vi "Teleop.vi"(10 "Match Info":T1={"Autonomous Elapsed Seconds"=0.0, "TeleOp Elapsed Seconds"=0.0, "Disabled Elapsed Seconds"=0.0, "Visited Autonomous"=FALSE, "Visited TeleOp"=FALSE, "Visited Disabled"=FALSE, "Autonomous Settings"={"Autonomous Style"=enum."Independent", "VI Refnum"=refnum}}, 11 "Call Context":T2) -> ()   [LabVIEW 2012]
doc: "This VI is called for each TeleOp packet received from the DS where the robot is not disabled. It is often used to read from the joysticks and update I/O or to update setpoints for timed control loops. It should complete and return within 20 milliseconds or it may miss DS packets."
uses:
  <vilib>/Rock Robotics/WPI/DriverStation/WPI_DriverStationDerivedRobotMode.ctl
  <vilib>/Rock Robotics/WPI/DriverStation/WPI_DriverStationMatch Info.ctl
  <vilib>/Rock Robotics/WPI/Relay/WPI_RelayValue.ctl
  Robot Global Data.vi
  <vilib>/Rock Robotics/WPI/Joystick/WPI_JoystickGetSetRefNum.vi
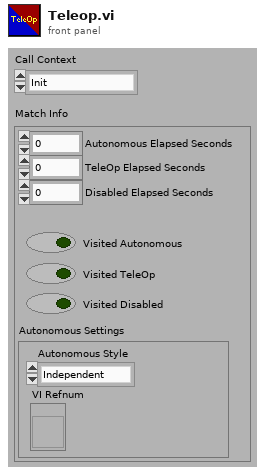
[diagram p1: front panel]
types:
  T1 = typedef "WPI_DriverStationMatch Info.ctl" = cluster{"Autonomous Elapsed Seconds":dbl, "TeleOp Elapsed Seconds":dbl, "Disabled Elapsed Seconds":dbl, "Visited Autonomous":bool, "Visited TeleOp":bool, "Visited Disabled":bool, "Autonomous Settings":cluster{"Autonomous Style":enum16{"Iterative", "Independent"}, "VI Refnum":refnum<vi>}}
  T2 = typedef "WPI_DriverStationDerivedRobotMode.ctl" = enum16{"Init", "Execute", "Stop"}
  T3 = typedef "WPI_JoystickDevRef.ctl" = cluster{"Device":T4}
  T4 = typedef "WPI_JoystickDeviceEnum.ctl" = enum16{"USB 1", "USB 2", "USB 3", "USB 4", "Kinect 1", "Kinect 2"}
  T5 = typedef "WPI_JoystickButtonState.ctl" = cluster{"Button 1":bool, "Button 2":bool, "Button 3":bool, "Button 4":bool, "Button 5":bool, "Button 6":bool, "Button 7":bool, "Button 8":bool, "Button 9":bool, "Button 10":bool, "Button 11":bool, "Button 12":bool}
  T6 = cluster{"axis 1 (x)":dbl, "axis 2 (y)":dbl, "axis 3 (throttle)":dbl, "axis 4":dbl, "axis 5":dbl, "axis 6":dbl}
  T7 = typedef "WPI_RelayValue.ctl" = enum16{"Off", "On", "Forward", "Reverse"}
  T8 = typedef "WPI_MotorControlDeviceRef.ctl" = cluster{"DeviceStatus":errorcluster, "Type":enum16{"PWM", "CAN"}, "PWM":cluster{"Digital Module":T9, "PWM Channel":T10, "DeadBand":T11}, "CAN":cluster{"Device Number":u8, "Control Mode":T12, "Semaphore":T13, "Max Vout":dbl}, "Invert":bool, "TransformRef":T14, "InvTransformRef":T14}
  T9 = typedef "FPGA_TypedefDigitalModule.ctl" = enum16{"Digital Module 1", "Digital Module 2"}
  T10 = typedef "FPGA_DIOPWMChannel.ctl" = enum8{"PWM 1", "PWM 2", "PWM 3", "PWM 4", "PWM 5", "PWM 6", "PWM 7", "PWM 8", "PWM 9", "PWM 10", "Invalid"}
  T11 = typedef "WPI_PWMDeadband.ctl" = cluster{"Name":string, "maxPositivePwm":i32, "minPositivePwm":i32, "centerPwm":i32, "maxNegativePwm":i32, "minNegativePwm":i32, "angularRange":u16}
  T12 = typedef "WPI_CANJaguar_ControlMode.ctl" = enum8{"Percent VBus", "Current", "Speed", "Position", "Voltage"}
  T13 = typedef "Semaphore RefNum" = refnum<k1>
  T14 = typedef "WPI_PWMTransform_ConPane.ctl" = refnum<vi>
  T15 = typedef "WPI_RelayDevRef.ctl" = cluster{"DevStatus":errorcluster, "Relay Channel":T16, "Digital Module":T9, "Relay Direction":T17}
  T16 = typedef "FPGA_DIORelayChannel.ctl" = enum8{"Relay 1", "Relay 2", "Relay 3", "Relay 4", "Relay 5", "Relay 6", "Relay 7", "Relay 8", "Invalid"}
  T17 = typedef "WPI_RelayDirection.ctl" = enum16{"Both directions", "Forward only", "Reverse only"}
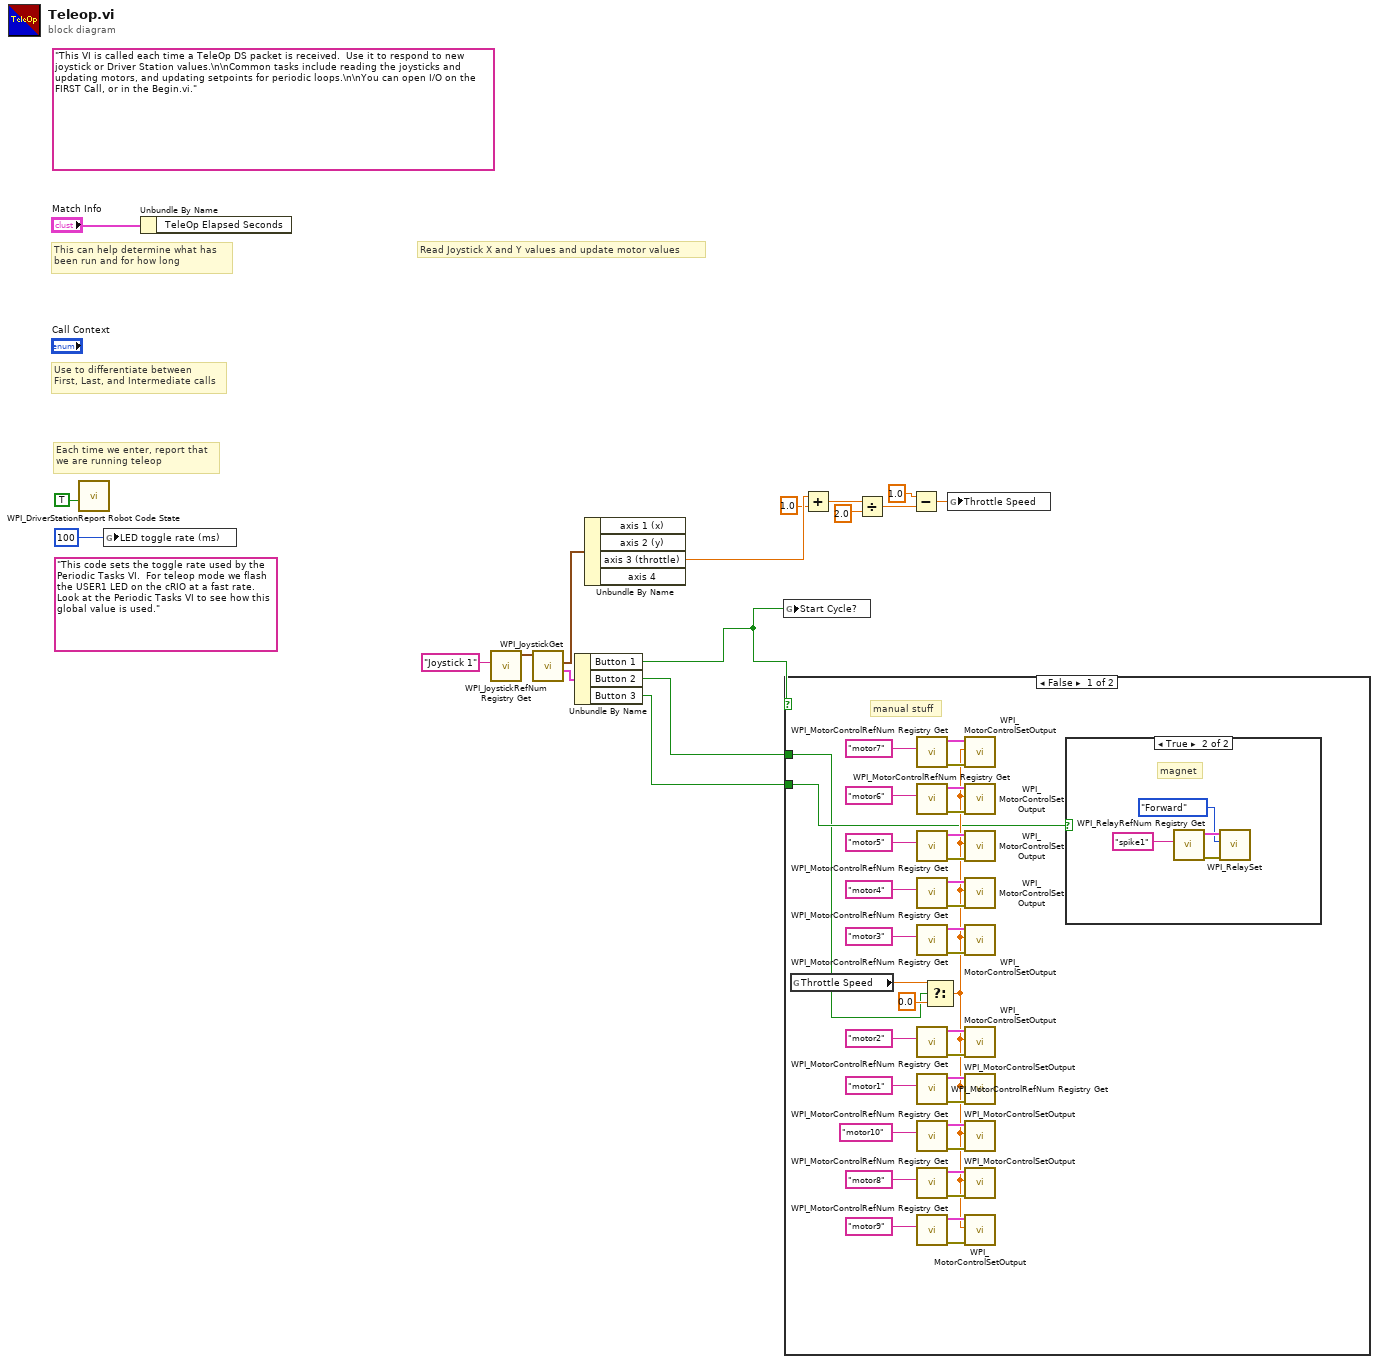
[diagram p0: block diagram]
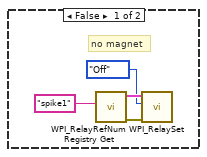
[diagram p2: hidden frame]
diagram:
  (unwired) "This code sets the toggle rate used by the Periodic Tasks VI.  For teleop mode we flash the USER1 LED on the cRIO at a fast rate.  Look at the Periodic Tasks VI to see how this global value is used."
  (unwired) "This VI is called each time a TeleOp DS packet is received.  Use it to respond to new joystick or Driver Station values.\n\nCommon tasks include reading the joysticks and updating motors, and updating setpoints for periodic loops.\n\nYou can open I/O on the FIRST Call, or in the Begin.vi."
  # "Each time we enter, report that\nwe are running teleop"
  # "Use to differentiate between\nFirst, Last, and Intermediate calls"
  # "This can help determine what has\nbeen run and for how long"
  # "Read Joystick X and Y values and update motor values"
  n1 = call <vilib>:"WPI_DriverStationReport Robot Code State.vi"("TeleOp"=TRUE ("Autonomous")) -> ()  [unwired: 10 in, 1 out]
  n2 = global write "Robot Global Data.vi" "LED toggle rate (ms)"(u32 100 ("LED ms toggle rate")) -> ()
  n3 = Unbundle By Name("Match Info") -> ()  [unwired: 1 out]
  n4 = call <vilib>:"WPI_JoystickRefNum Registry Get.vi"("refnum name"="Joystick 1") -> ("JoystickDevRef"=w15:T3)  [unwired: 1 in, 9 out]
  n5 = call <vilib>:"WPI_JoystickGet.vi"("JoystickDevRef"=w15) -> ("Buttons"=w12:T5, "Axes"=w8:T6)  [unwired: 1 in, 4 out]
  n6 = Unbundle By Name(w12) -> ("Button 1"=w9:bool, "Button 2"=w11:bool, "Button 3"=w10:bool)
  n7 = Unbundle By Name(w8) -> ("axis 3 (throttle)"=w7:dbl)  [unwired: 3 out]
  n8 = global write "Robot Global Data.vi" "Start Cycle?"(w9) -> ()
  n9 = case shown="False" w9 {
    tunnel: w11 -> [w19 _]
    tunnel: w10 -> [w20 _]
    frame False {
      # "manual stuff"
      n10 = global read "Robot Global Data.vi" "Throttle Speed"() -> (w18:dbl)
      n11 = call <vilib>:"WPI_MotorControlRefNum Registry Get.vi"("refnum name"="motor7") -> ("error out"=w40:errorcluster, "MotorControlDevRef"=w41:T8)  [unwired: 9 in]
      n12 = call <vilib>:"WPI_MotorControlRefNum Registry Get.vi"("refnum name"="motor6") -> ("error out"=w37:errorcluster, "MotorControlDevRef"=w38:T8)  [unwired: 9 in]
      n13 = call <vilib>:"WPI_MotorControlRefNum Registry Get.vi"("refnum name"="motor5") -> ("error out"=w34:errorcluster, "MotorControlDevRef"=w35:T8)  [unwired: 9 in]
      n14 = call <vilib>:"WPI_MotorControlRefNum Registry Get.vi"("refnum name"="motor4") -> ("error out"=w31:errorcluster, "MotorControlDevRef"=w32:T8)  [unwired: 9 in]
      n15 = call <vilib>:"WPI_MotorControlRefNum Registry Get.vi"("refnum name"="motor3") -> ("error out"=w28:errorcluster, "MotorControlDevRef"=w29:T8)  [unwired: 9 in]
      n16 = call <vilib>:"WPI_MotorControlRefNum Registry Get.vi"("refnum name"="motor2") -> ("error out"=w25:errorcluster, "MotorControlDevRef"=w26:T8)  [unwired: 9 in]
      n17 = call <vilib>:"WPI_MotorControlRefNum Registry Get.vi"("refnum name"="motor1") -> ("error out"=w22:errorcluster, "MotorControlDevRef"=w23:T8)  [unwired: 9 in]
      n18 = call <vilib>:"WPI_MotorControlRefNum Registry Get.vi"("refnum name"="motor10") -> ("error out"=w49:errorcluster, "MotorControlDevRef"=w50:T8)  [unwired: 9 in]
      n19 = call <vilib>:"WPI_MotorControlRefNum Registry Get.vi"("refnum name"="motor8") -> ("error out"=w43:errorcluster, "MotorControlDevRef"=w44:T8)  [unwired: 9 in]
      n20 = call <vilib>:"WPI_MotorControlRefNum Registry Get.vi"("refnum name"="motor9") -> ("error out"=w46:errorcluster, "MotorControlDevRef"=w47:T8)  [unwired: 9 in]
      n21 = Select(t=w18, s=w19, f=0.0) -> (s? t:f=w21:dbl)
      n22 = call <vilib>:"WPI_MotorControlSetOutput.vi"("error in (no error)"=w40, "Output"=w21, "MotorControlDevRef"=w41) -> ()  [unwired: 6 in, 3 out]
      n23 = call <vilib>:"WPI_MotorControlSetOutput.vi"("error in (no error)"=w37, "Output"=w21, "MotorControlDevRef"=w38) -> ()  [unwired: 6 in, 3 out]
      n24 = call <vilib>:"WPI_MotorControlSetOutput.vi"("error in (no error)"=w34, "Output"=w21, "MotorControlDevRef"=w35) -> ()  [unwired: 6 in, 3 out]
      n25 = call <vilib>:"WPI_MotorControlSetOutput.vi"("error in (no error)"=w31, "Output"=w21, "MotorControlDevRef"=w32) -> ()  [unwired: 6 in, 3 out]
      n26 = call <vilib>:"WPI_MotorControlSetOutput.vi"("error in (no error)"=w28, "Output"=w21, "MotorControlDevRef"=w29) -> ()  [unwired: 6 in, 3 out]
      n27 = call <vilib>:"WPI_MotorControlSetOutput.vi"("error in (no error)"=w25, "Output"=w21, "MotorControlDevRef"=w26) -> ()  [unwired: 6 in, 3 out]
      n28 = call <vilib>:"WPI_MotorControlSetOutput.vi"("error in (no error)"=w22, "Output"=w21, "MotorControlDevRef"=w23) -> ()  [unwired: 6 in, 3 out]
      n29 = call <vilib>:"WPI_MotorControlSetOutput.vi"("error in (no error)"=w49, "Output"=w21, "MotorControlDevRef"=w50) -> ()  [unwired: 6 in, 3 out]
      n30 = call <vilib>:"WPI_MotorControlSetOutput.vi"("error in (no error)"=w43, "Output"=w21, "MotorControlDevRef"=w44) -> ()  [unwired: 6 in, 3 out]
      n31 = call <vilib>:"WPI_MotorControlSetOutput.vi"("error in (no error)"=w46, "Output"=w21, "MotorControlDevRef"=w47) -> ()  [unwired: 6 in, 3 out]
      n32 = case shown="True" w20 {
        frame False {
          # "no magnet"
          n33 = call <vilib>:"WPI_RelayRefNum Registry Get.vi"("refnum name"="spike1") -> ("error out"=w56:errorcluster, "RelayDevRef"=w55:T15)  [unwired: 9 in]
          n34 = call <vilib>:"WPI_RelaySet.vi"("error in (no error)"=w56, "RelayValue"=WPI_RelayValue."Off", "RelayDevRef"=w55) -> ()  [unwired: 7 in, 2 out]
        }
        frame True {
          # "magnet"
          n35 = call <vilib>:"WPI_RelayRefNum Registry Get.vi"("refnum name"="spike1") -> ("error out"=w60:errorcluster, "RelayDevRef"=w59:T15)  [unwired: 9 in]
          n36 = call <vilib>:"WPI_RelaySet.vi"("error in (no error)"=w60, "RelayValue"=WPI_RelayValue."Forward", "RelayDevRef"=w59) -> ()  [unwired: 7 in, 2 out]
        }
      }
    }
    frame True {
      # "run sequenced code"
    }
  }
  n37 = Add(x=w7, y=1.0) -> (x+y=w5:dbl)
  n38 = Divide(x=w5, y=2.0) -> (x/y=w3:dbl)
  n39 = Subtract(x=1.0, y=w3) -> (x-y=w1:dbl)
  n40 = global write "Robot Global Data.vi" "Throttle Speed"(w1) -> ()
